vi "SubVIexamplefilesaving.vi"() -> ()   [LabVIEW 2018]
uses:
  Global Variables.vi
panel:
  in  "stop":bool
  in  "Save Data TDMS":bool
  out "Independent?":bool
  in  "Tab Control":enum32{"File", "Setup"}(tab)=enum."Setup"
  out "Filepath":path=path "C:/Labview Test Data/2018-08-07/0/Temp Dependence/Sensors_DAQ_200C_2.tdms"
  out "VI name":string="Sensors_DAQ"
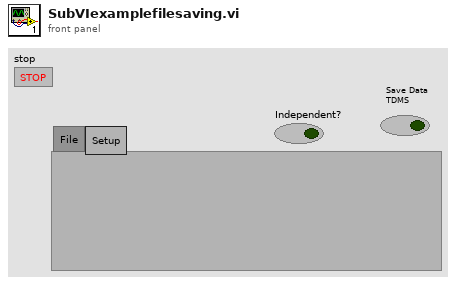
[diagram p1: front panel]
types:
  T1 = cluster{"Project":u16, "SubFolder":string, "Filename (Meas. Description)":string, "Measurement index":i32}
  T2 = cluster{"Ring":u16, "SubFolder":string, "Filename (Meas. Description)":string, "Measurement index":i32}
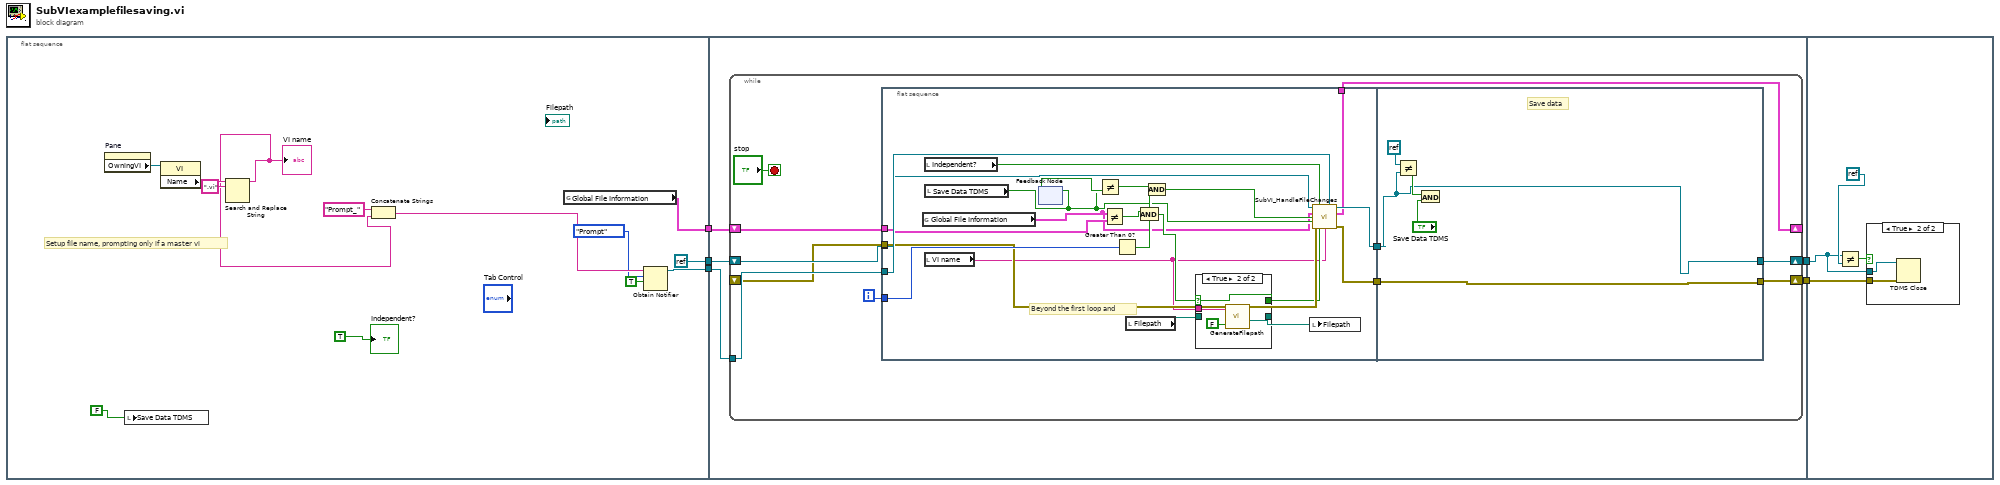
[diagram p0: block diagram]
diagram:
  n1 = flat-sequence {
    tunnel: [w10] -> w5
    tunnel: [refnum<k0> refnum] -> w2
    tunnel: [w6] -> w1
    tunnel: w5 -> [w23]
    tunnel: [w22] -> w4
    tunnel: [w21] -> w3
    tunnel: w2 -> [w20]
    tunnel: w1 -> [w19]
    tunnel: w4 -> [w70]
    tunnel: w3 -> [w67]
    frame #0 {
      # "Setup file name, prompting only if a master vi"
      n2 = property on="Pane" class="Pane"() -> ("OwningVI"=w18:refnum<vi>)  [unwired: 2 in, 2 out]
      n3 = local write "Save Data TDMS"(FALSE) -> ()
      n4 = property class="VI"(reference=w18) -> ("Name"=w17:string)  [unwired: 1 in, 2 out]
      n5 = Search and Replace String(input string=w17, search string=".vi") -> (result string=w8:string)  [unwired: 6 in, 3 out]
      "VI name" <- w8
      n6 = Concatenate Strings("Prompt_" ("string"), w8) -> (w13:string)
      n7 = global read "Global Variables.vi" "Global File Information"() -> (w6:T1)
      n8 = Obtain Notifier(name (unnamed)=w13, notification data type=enum16{"Prompt", "Keep", "Archive", "Trash"}."Prompt" ("Action"), create if not found? (T)=TRUE) -> (notifier out=w10:refnum<notifier>)  [unwired: 1 in, 2 out]
      "Independent?" <- TRUE ("Independent?")
    }
    frame #1 {
      n9 = while {
        tunnel: w23 -> [w33]
        shift-right: [w27] -> w21
        shift-left: w20 -> [w32]
        shift-right: [w28] -> w22
        shift-left: _ -> [w31]
        shift-right: [w25] -> _
        shift-left: w19 -> [w26]
        i -> [w34]
        stop <- "stop" stop-if-true
        n10 = flat-sequence {
          tunnel: w34 -> [w53]
          tunnel: w33 -> [w55]
          tunnel: w32 -> [w48]
          tunnel: w31 -> [w47]
          tunnel: [w46] -> w30
          tunnel: [w45] -> w29
          tunnel: w26 -> [w37]
          tunnel: [w35] -> w25
          tunnel: w30 -> [w62]
          tunnel: w29 -> [w63]
          tunnel: [w63] -> w28
          tunnel: [w62] -> w27
          frame #0 {
            # "Beyond the first loop and"
            n11 = global read "Global Variables.vi" "Global File Information"() -> (w36:T1)
            n12 = local read "Independent?"() -> (w40:bool)
            n13 = local read "VI name"() -> (w38:string)
            n14 = local read "Save Data TDMS"() -> (w39:bool)
            n15 = feedback #1() -> (w52:bool)  [unwired: 1 in]
            n16 = feedback-in #1(w39) -> ()
            n17 = Not Equal?(x=w52, y=w39) -> (x != y?=w51:bool)
            n18 = Not Equal?(x=w36, y=w37) -> (x != y?=w54:bool)
            n19 = Greater Than 0?(x=w53) -> (x > 0?=w50:bool)
            n20 = local read "Filepath"() -> (w42:path)
            n21 = Compound Arithmetic op=AND(w54, w50) -> (w44:bool)
            n22 = Compound Arithmetic op=AND(w51, w50) -> (w49:bool)
            n23 = case shown="True" w44 {
              selector: w44 -> [w56 w61]
              tunnel: [w56 w61] -> w43
              tunnel: w42 -> [w57 _]
              tunnel: [w57 w60] -> w41
              tunnel: w38 -> [_ w59]
              frame False {
              }
              frame True {
                n24 = call "GenerateFilepath.vi"("Instrument"=w59, "Check for file?"=FALSE) -> ("File Path Out"=w60:path)  [unwired: 3 in, 1 out]
              }
            }
            n25 = local write "Filepath"(w41) -> ()
            n26 = call "SubVI_HandleFileChanges.vi"("File Refnum in"=w48, "Independent?"=w40, "notifier in"=w55, "Global File Information"=w36, "Sava data tured on or off?"=w49, "Save Data TDMS"=w39, "error in (no error)"=w47, "File Info Changed?"=w43, "VI name"=w38) -> ("File Refnum out"=w46:refnum<k34>, "Global File Information out"=w35:T2, "error out"=w45:errorcluster)  [unwired: 4 in]
          }
          frame #1 {
            # "Save data"
            n27 = Not Equal?(x=refnum<k0> refnum, y=w62) -> (x != y?=w66:bool)
            n28 = And(x=w66, y="Save Data TDMS") -> ()  [unwired: 1 out]
          }
        }
      }
    }
    frame #2 {
      n29 = Not Equal?(x=w67, y=refnum<k0> refnum) -> (x != y?=w69:bool)
      n30 = case shown="True" w69 {
        tunnel: w70 -> [_ w72]
        tunnel: w67 -> [_ w71]
        frame False {
        }
        frame True {
          n31 = TDMS Close(8:w72, 11:w71) -> ()  [unwired: 2 out]
        }
      }
    }
  }
